vi "Realtime Clock-Remote.vi"() -> ()   [LabVIEW 2009]
uses:
  <vilib>/NXT/Subs/LVHSConnector.ctl
  <vilib>/NXT/Block Support/NXT_InputPort.ctl
panel:
  in  "Input Port":T1 items=["Port 1", "Port 2", "Port 3", "Port 4"]
  out "NXT dup":T2
  in  "NXT":T2
  # "mindsensors.com\nCopyright (c) 2009 by mindsensors.com\nEmail: info (<at>) mindsensors (<dot>) com\n\nThis program is free software. You can redistribute it and/or modify\nit under the terms of the GNU General Public License as published by\nthe Free Software Foundation; version 3 of the License.\nRead the license at: http://www.gnu.org/licenses/gpl.txt"
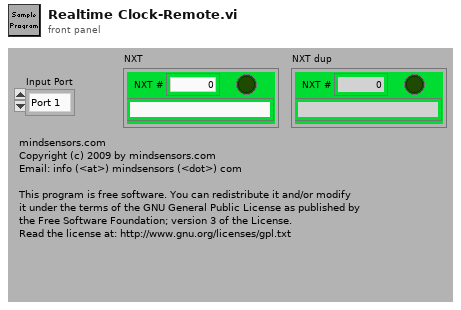
[diagram p1: front panel]
types:
  T1 = typedef "NXT_InputPort.ctl" = u8
  T2 = typedef "LVHSConnector.ctl" = cluster{"error":errorcluster, "address":string, "NXT #":i32, "Show Error":bool}
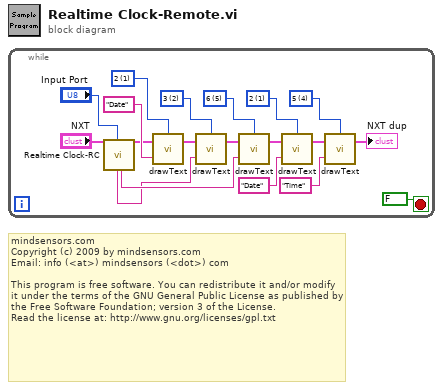
[diagram p0: block diagram]
diagram:
  # "mindsensors.com\nCopyright (c) 2009 by mindsensors.com\nEmail: info (<at>) mindsensors (<dot>) com\n\nThis program is free software. You can redistribute it and/or modify\nit under the terms of the GNU General Public License as published by\nthe Free Software Foundation; version 3 of the License.\nRead the license at: http://www.gnu.org/licenses/gpl.txt"
  n1 = while {
    stop <- FALSE stop-if-true
    w12 = i16 1 items=["1", "2", "3", "4", "5", "6", "7", "8"] ("Line")
    w15 = i16 4 items=["1", "2", "3", "4", "5", "6", "7", "8"] ("Line")
    w17 = i16 1 items=["1", "2", "3", "4", "5", "6", "7", "8"] ("Line")
    w18 = i16 2 items=["1", "2", "3", "4", "5", "6", "7", "8"] ("Line")
    w19 = i16 5 items=["1", "2", "3", "4", "5", "6", "7", "8"] ("Line")
    n2 = call "Realtime Clock-RC.vi"("NXT"="NXT", "Input Port"="Input Port") -> ("date string"=w9:string, "time string"=w10:string, "NXT dup"=w7:T2)  [unwired: 16 in, 7 out]
    n3 = call <vilib>:"drawText.vi"("Text"="Date", "NXT"=w7, "Line"=w12) -> ("NXT"=w6:T2)  [unwired: 1 in]
    n4 = call <vilib>:"drawText.vi"("Text"=w9, "NXT"=w6, "Line"=w18) -> ("NXT"=w5:T2)  [unwired: 1 in]
    n5 = call <vilib>:"drawText.vi"("Text"=w10, "NXT"=w5, "Line"=w19) -> ("NXT"=w4:T2)  [unwired: 1 in]
    n6 = call <vilib>:"drawText.vi"("Text"="Date", "NXT"=w4, "Line"=w17) -> ("NXT"=w3:T2)  [unwired: 1 in]
    n7 = call <vilib>:"drawText.vi"("Text"="Time", "NXT"=w3, "Line"=w15) -> ("NXT"=→"NXT dup":T2)  [unwired: 1 in]
  }
